vi "FIR.vi"() -> ()   [LabVIEW 2015]
uses:
  <vilib>/sound2/lvsound2.llb/Sound Data Format.ctl
  <vilib>/sound2/lvsound2.llb/Sound File Info (path).vi
panel:
  out "1/x":dbl
  out "dt":dbl
  in  "FIR Coefficients 3":dbl[](array[numeric])
  out "Time-Domain 5":waveform(dbl)(graph)
  out "Spectrum 5":cluster{"f0":dbl, "df":dbl, "magnitude":dbl[]}(graph)
  in  "FIR Coefficients 2":dbl[](array[numeric])
  out "Time-Domain 4":waveform(dbl)(graph)
  out "Spectrum 4":cluster{"f0":dbl, "df":dbl, "magnitude":dbl[]}(graph)
  in  "FIR Coefficients":dbl[](array[numeric])
  out "Time-Domain 3":waveform(dbl)(graph)
  out "Spectrum 3":cluster{"f0":dbl, "df":dbl, "magnitude":dbl[]}(graph)
  out "Time-Domain 2":waveform(dbl)(graph)
  out "Spectrum 2":cluster{"f0":dbl, "df":dbl, "magnitude":dbl[]}(graph)
  out "sound format":T1={"sample rate (S/s)"=22050.0, "number of channels"=2, "bits per sample"=16}
  in  "fc":dbl
  out "Time-Domain":waveform(dbl)(graph)
  out "Spectrum":cluster{"f0":dbl, "df":dbl, "magnitude":dbl[]}(graph)
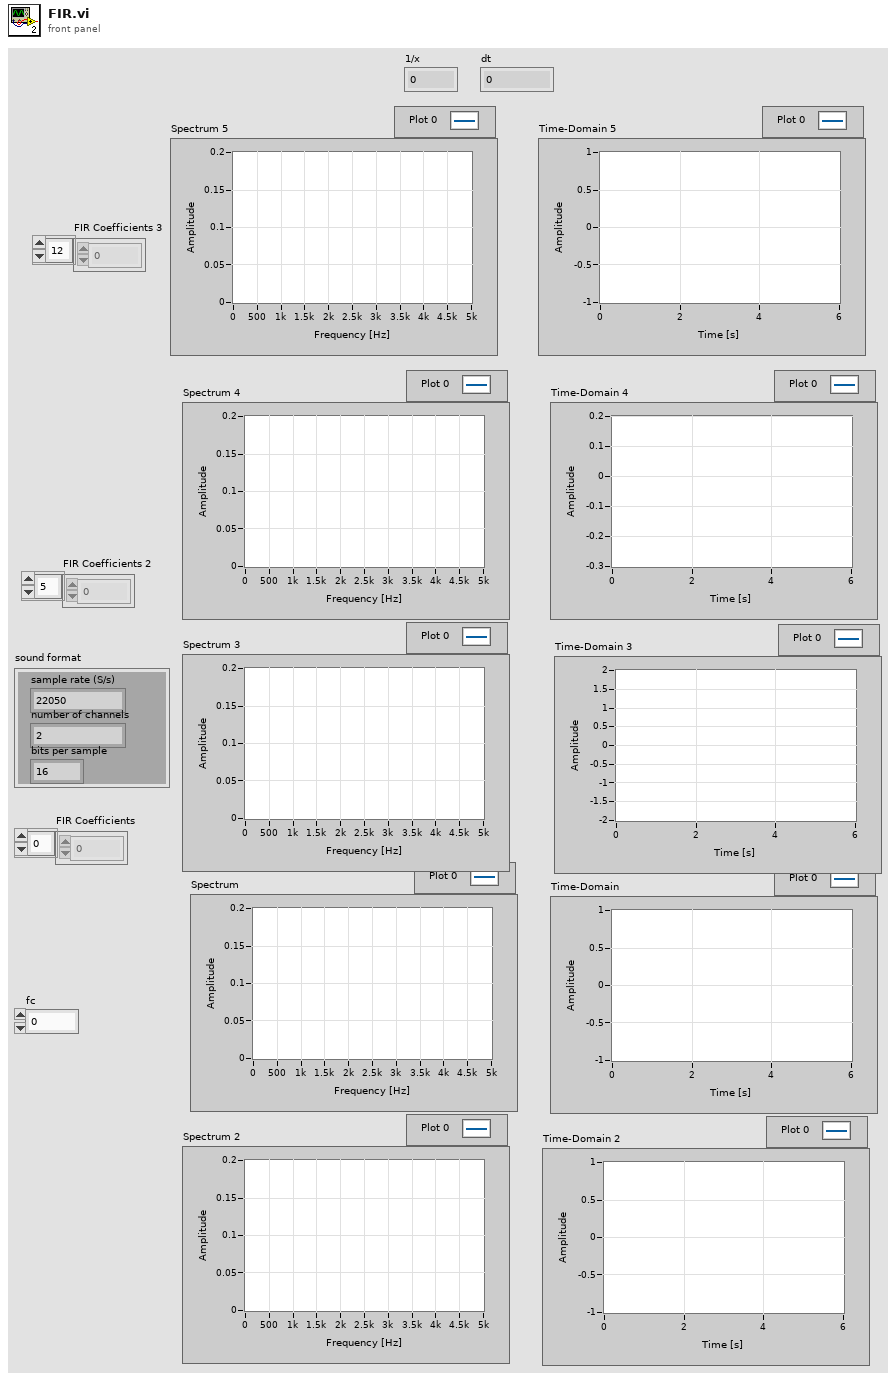
[diagram p1: front panel]
types:
  T1 = typedef "Sound Data Format.ctl" = cluster{"sample rate (S/s)":dbl, "number of channels":i32, "bits per sample":i32}
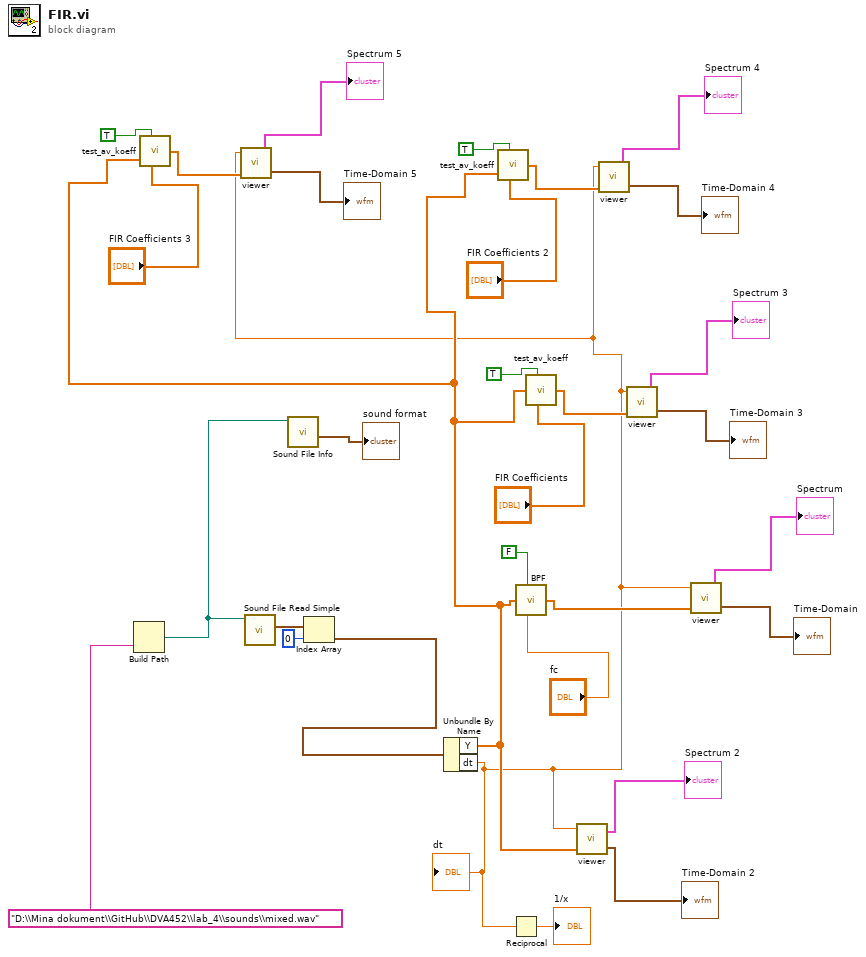
[diagram p0: block diagram]
diagram:
  n1 = Build Path(name or relative path="D:\\Mina dokument\\GitHub\\DVA452\\lab_4\\sounds\\mixed.wav") -> (appended path=w24:path)  [unwired: 1 in]
  n2 = call <vilib>:"Sound File Read Simple.vi"("path"=w24) -> ("data"=w29:waveform(dbl)[])  [unwired: 7 in, 3 out]
  n3 = call-poly <vilib>:"Sound File Info.vi"("path"=w24) -> ("sound format"=→"sound format":T1)  [unwired: 7 in, 3 out]
  n4 = Index Array(array=w29, index=0) -> (element=w27:waveform(dbl))
  n5 = Unbundle By Name(w27) -> ("Y"=w3:dbl[], "dt"=w2:dbl)
  "dt" <- w2
  n6 = call "test_av_koeff.vi"("s"=TRUE ("enable"), "in"=w3, "FIR Coefficients"="FIR Coefficients 3") -> ("out"=w5:dbl[])  [unwired: 4 in]
  n7 = call "viewer.vi"("in"=w5, "f_s"=w2) -> ("Time-Domain"=→"Time-Domain 5":waveform(dbl), "Spectrum"=→"Spectrum 5":cluster{"f0":dbl, "df":dbl, "magnitude":dbl[]})  [unwired: 1 in]
  n8 = call "test_av_koeff.vi"("s"=TRUE ("enable"), "in"=w3, "FIR Coefficients"="FIR Coefficients 2") -> ("out"=w10:dbl[])  [unwired: 4 in]
  n9 = Reciprocal(x=w2) -> (1/x=→"1/x":dbl)
  n10 = call "BPF.vi"("enable"=FALSE, "in"=w3, "fc"="fc") -> ("out"=w19:dbl[])  [unwired: 4 in]
  n11 = call "test_av_koeff.vi"("s"=TRUE ("enable"), "in"=w3, "FIR Coefficients"="FIR Coefficients") -> ("out"=w15:dbl[])  [unwired: 4 in]
  n12 = call "viewer.vi"("in"=w3, "f_s"=w2) -> ("Time-Domain"=→"Time-Domain 2":waveform(dbl), "Spectrum"=→"Spectrum 2":cluster{"f0":dbl, "df":dbl, "magnitude":dbl[]})  [unwired: 1 in]
  n13 = call "viewer.vi"("in"=w10, "f_s"=w2) -> ("Time-Domain"=→"Time-Domain 4":waveform(dbl), "Spectrum"=→"Spectrum 4":cluster{"f0":dbl, "df":dbl, "magnitude":dbl[]})  [unwired: 1 in]
  n14 = call "viewer.vi"("in"=w15, "f_s"=w2) -> ("Time-Domain"=→"Time-Domain 3":waveform(dbl), "Spectrum"=→"Spectrum 3":cluster{"f0":dbl, "df":dbl, "magnitude":dbl[]})  [unwired: 1 in]
  n15 = call "viewer.vi"("in"=w19, "f_s"=w2) -> ("Time-Domain"=→"Time-Domain":waveform(dbl), "Spectrum"=→"Spectrum":cluster{"f0":dbl, "df":dbl, "magnitude":dbl[]})  [unwired: 1 in]
